vi "LoadProjectData.vi"(8 "error in (no error)":errorcluster, 11 "MPC_VirbVision in":refnum<class "MPC_VirbVision.lvclass">) -> (0 "error out":errorcluster, 3 "MPC_VirbVision out":refnum<class "MPC_VirbVision.lvclass">)   [LabVIEW 2019, in "MPC_VirbVision.lvclass"]
uses:
  MPC_VirbVision.lvclass
  Function/20200219Virbtion/Typedef/State.ctl
  LLB/Commonly VI/Ctrl/IDLevel.ctl
  Panel RefGlb.vi
  LLB/Commonly VI/Load Glb.vi
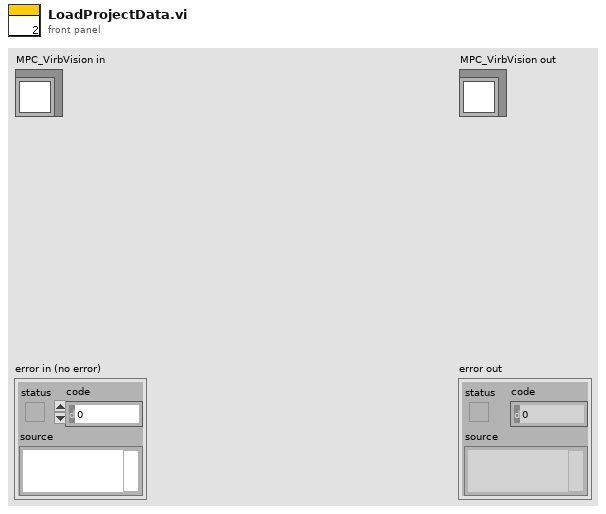
[diagram p1: front panel]
types:
  T1 = enum16{"initial", "save", "load", "write", "read"}
  T2 = enum16{"Initial", "Load", "Save", "Read", "WriteSpeed", "WritePoint"}
  T3 = enum8{"Enabled", "Disabled", "Disabled and Grayed Out"}
  T4 = typedef "IDLevel.ctl" = enum16{"Administrator", "Engineer", "Operator", "LogIn/Out"}
  T5 = typedef "State.ctl" = enum16{"Initalize", "Idle", "Update", "Channel1", "Channel2", "Channel3", "Channel4", "Channel1 Sample", "Channel2 Sample", "Channel3 Sample", "Channel4 Sample", "Waveform", "DAQ Rate", "ModelList", "Add", "Remove", "Set Time", "Test", "Start Time", "Check Time", "Save", "Frontward", "Leftward", "Backward", "Rightward", "Stop", "Center", "Bump", "Add Project", "Remove Project", "Project List", "Project Name", "Project OK", "Response", "Exit"}
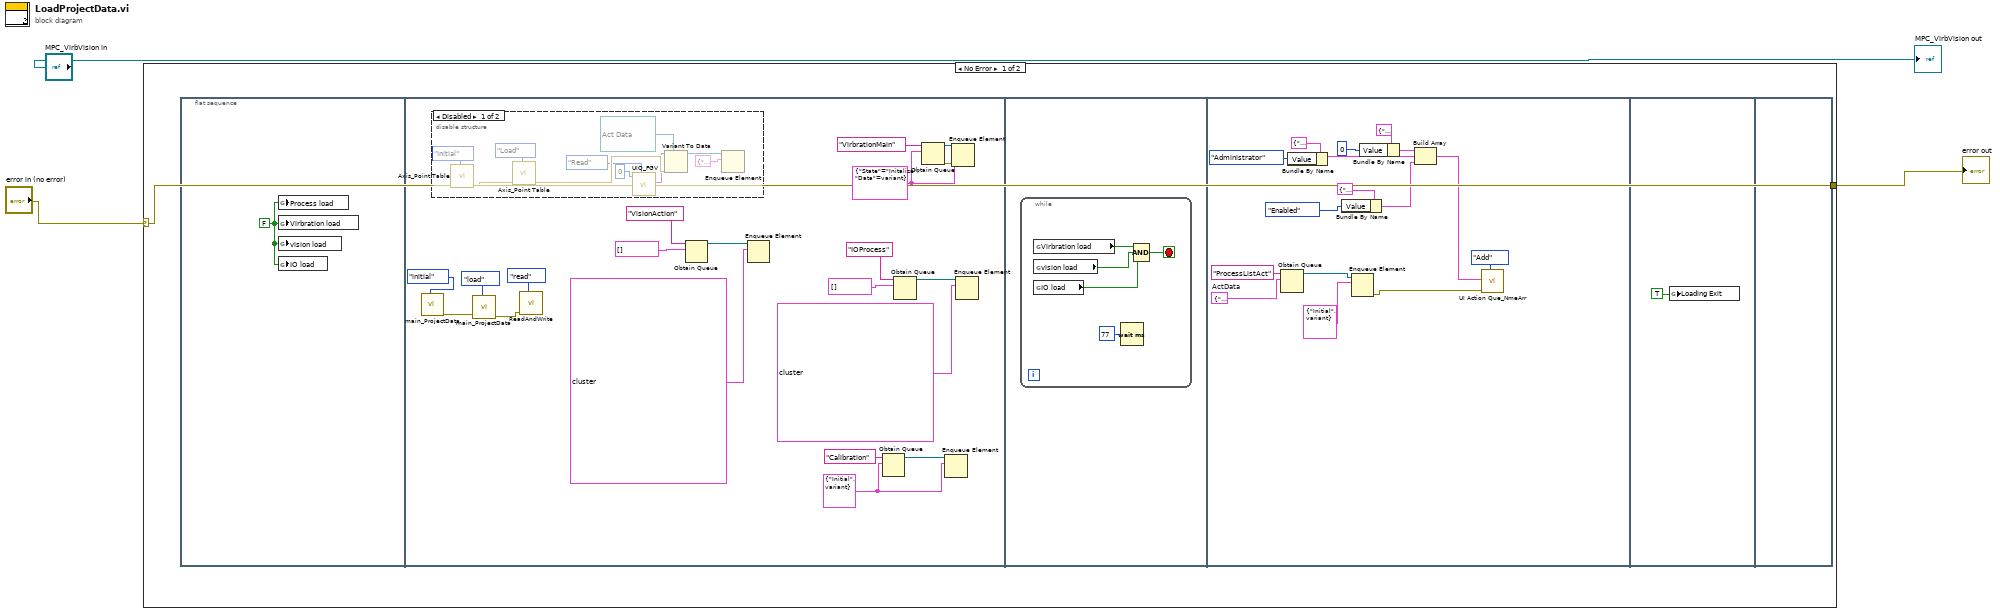
[diagram p0: block diagram]
diagram:
  n1 = case shown="No Error" "error in (no error)" {
    selector: "error in (no error)" -> [w4 w58]
    tunnel: [w4 w58] -> w2
    frame No Error {
      n2 = flat-sequence {
        frame #0 {
          w5 = FALSE ("IO load")
          n3 = global write "Panel RefGlb.vi" "Process load"(w5) -> ()
          n4 = global write "Panel RefGlb.vi" "Virbration load"(w5) -> ()
          n5 = global write "Panel RefGlb.vi" "vision load"(w5) -> ()
          n6 = global write "Panel RefGlb.vi" "IO load"(w5) -> ()
        }
        frame #1 {
          w22 = cluster{"State":T5, "Data":variant} {"State"=enum."Initalize", "Data"=variant}
          w23 = cluster{"Action":string, "Varient":variant} {"Action"="Initial", "Varient"=variant} ("element")
          n7 = call "main_ProjectData.vi"("Enum"=T1."initial") -> ("error out"=w6:errorcluster)  [unwired: 8 in, 2 out]
          n8 = disable-structure shown="Disabled" {
            frame Disabled {
              n9 = call "Axis_Point Table.vi"("Enum"=T2."Initial") -> ("error Out"=w35:errorcluster)  [unwired: 8 in, 2 out]
              n10 = call "Axis_Point Table.vi"("Enum"=T2."Load", "error In"=w35) -> ("error Out"=w33:errorcluster)  [unwired: 7 in, 2 out]
              n11 = call "UIQ_FGV.vi"("Enum"=enum16{"Initial", "Write", "Read"}."Read", "Index"=0) -> ("DataOut"=w29:variant)  [unwired: 9 in]
              n12 = Variant To Data(error in=w33, type=refnum<queue> refnum ("Axis Q"), Variant=w29) -> (data=w30:refnum<queue>)  [unwired: 1 out]
              n13 = Enqueue Element(queue=w30, element=cluster{"Action":string, "Data":variant} {"Action"="LoadParameter", "Data"=variant}) -> ()  [unwired: 2 in, 3 out]
            }
            frame Enabled {
            }
          }
          n14 = call "main_ProjectData.vi"("Enum"=T1."load", "error in"=w6) -> ("error out"=w10:errorcluster)  [unwired: 7 in, 2 out]
          n15 = call "ReadAndWrite.vi"("Enum"=enum16{"initial", "save", "read"}."read", "error in"=w10) -> ()  [unwired: 9 in, 1 out]
          n16 = Obtain Queue(name (unnamed)="VisionAction", element data type=cluster{"Action":string, "Varient":variant}[] []) -> (queue out=w12:refnum<queue>)  [unwired: 3 in, 2 out]
          n17 = Enqueue Element(queue=w12, element=cluster{"Action":string, "Varient":variant}[] [{"Action"="Get Root Path", "Varient"=variant}, {"Action"="Initial Project", "Varient"=variant}, {"Action"="UpdateProjectSet", "Varient"=variant}, {"Action"="UpDateDataToList ROI", "Varient"=variant}, {"Action"="Initial Camera", "Varient"=variant}, {"Action"="loadfinish", "Varient"=variant}]) -> ()  [unwired: 2 in, 3 out]
          n18 = Obtain Queue(name (unnamed)="Calibration", element data type=w23) -> (queue out=w24:refnum<queue>)  [unwired: 3 in, 2 out]
          n19 = Obtain Queue(name (unnamed)="IOProcess", element data type=cluster{"Action":string, "Varient":variant}[] []) -> (queue out=w16:refnum<queue>)  [unwired: 3 in, 2 out]
          n20 = Obtain Queue(name (unnamed)="VirbrationMain", element data type=w22) -> (queue out=w20:refnum<queue>, error out=w19:errorcluster)  [unwired: 3 in, 1 out]
          n21 = Enqueue Element(queue=w24, element=w23) -> ()  [unwired: 2 in, 3 out]
          n22 = Enqueue Element(queue=w20, element=w22, error in (no error)=w19) -> ()  [unwired: 1 in, 3 out]
          n23 = Enqueue Element(queue=w16, element=cluster{"Action":string, "Varient":variant}[] [{"Action"="Get Root Path", "Varient"=variant}, {"Action"="Initial Project", "Varient"=variant}, {"Action"="UpdateProjectSet", "Varient"=variant}, {"Action"="Initial IOName", "Varient"=variant}, {"Action"="loadfinish", "Varient"=variant}]) -> ()  [unwired: 2 in, 3 out]
        }
        frame #2 {
          n24 = while {
            stop <- w37 stop-if-true
            n25 = global read "Panel RefGlb.vi" "Virbration load"() -> (w40:bool)
            n26 = global read "Panel RefGlb.vi" "vision load"() -> (w39:bool)
            n27 = global read "Panel RefGlb.vi" "IO load"() -> (w38:bool)
            n28 = Wait (ms)(milliseconds to wait=u32 77) -> ()  [unwired: 1 out]
            n29 = Compound Arithmetic op=AND(w40, w39, w38) -> (w37:bool)
          }
        }
        frame #3 {
          w55 = cluster{"Action":string, "Data":variant} {"Action"="", "Data"=variant}  # ActData
          n30 = Obtain Queue(name (unnamed)="ProcessListAct", element data type=w55) -> (queue out=w53:refnum<queue>)  [unwired: 3 in, 2 out]
          n31 = Bundle By Name(cluster=cluster{"Action":string, "Value":variant} {"Action"="ChangeMenuBar", "Value"=variant} ("UI Action"), "Value"=IDLevel."Administrator" ("Entry Level")) -> (w44:cluster{"Action":string, "Value":variant})
          n32 = Bundle By Name(cluster=cluster{"Action":string, "Value":variant} {"Action"="AutorunEnable", "Value"=variant} ("UI Action"), "Value"=T3."Enabled" ("Disabled")) -> (w42:cluster{"Action":string, "Value":variant})
          n33 = Enqueue Element(queue=w53, element=cluster{"Action":string, "Data":variant} {"Action"="Initial", "Data"=variant}) -> (error out=w48:errorcluster)  [unwired: 2 in, 2 out]
          n34 = Bundle By Name(cluster=cluster{"Action":string, "Value":variant} {"Action"="ChangePage", "Value"=variant} ("UI Action"), "Value"=0) -> (w50:cluster{"Action":string, "Value":variant})
          n35 = Build Array(w50, w44, w42) -> (w49:cluster{"Action":string, "Value":variant}[])
          n36 = call "UI Action Que_NmeArr.vi"("Action"=enum16{"Initial", "Add", "Release"}."Add", "error in (no error)"=w48, "UI Process"=w49) -> ()  [unwired: 7 in, 2 out]
        }
        frame #4 {
          n37 = global write "Load Glb.vi" "Loading Exit"(TRUE ("Loading Exit")) -> ()
        }
        frame #5 {
        }
      }
    }
    frame Error {
    }
  }
  "error out" <- w2
  "MPC_VirbVision out" <- "MPC_VirbVision in"
